vi "Target Reset Running Trajectories.vi"(8 "Error":dbl, 11 "Phase":dbl) -> (0 "Running Error":dbl[](array[numeric]), 3 "Running Phase":dbl[](array[numeric]), 5 "index":i32)   [LabVIEW 2018, in "COBRA Iterative Learning Control Library.lvlib"]
uses:
  COBRA Iterative Learning Control Library.lvlib
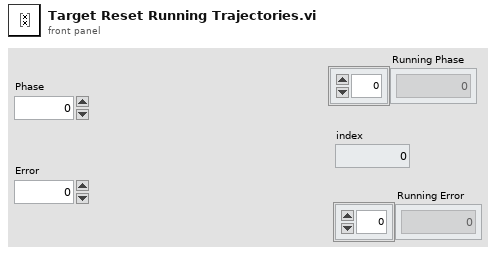
[diagram p1: front panel]
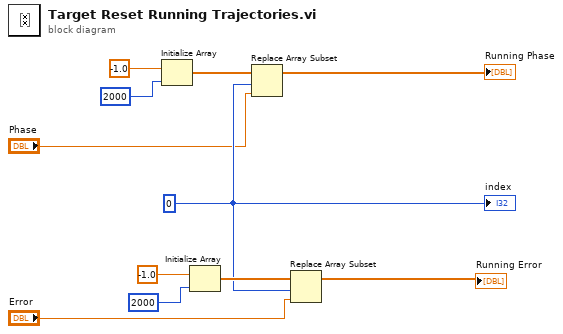
[diagram p0: block diagram]
diagram:
  w4 = 0 ("index")
  n1 = Initialize Array "Initialize Array"(-1.0 ("element"), 2000 ("dimension size")) -> (w7:dbl[])
  n2 = Initialize Array(-1.0 ("element"), 2000 ("dimension size")) -> (w6:dbl[])
  n3 = Replace Array Subset "Replace Array Subset"(array=w7, new element="Phase", index=w4) -> (→"Running Phase":dbl[])
  n4 = Replace Array Subset(array=w6, new element="Error", index=w4) -> (→"Running Error":dbl[])
  "index" <- w4
